vi "Load Table.vi"(4 "XY Graph2":refnum<vi>, 5 "XY Graph1":refnum<vi>, 6 "2 Mics? (F)":bool, 7 "Table Ref":refnum<vi>, 8 "error in (no error)":errorcluster, 9 "Result Cluster":T1, 10 "Config Type":T2={"PSU"={"Current Lower (mA)"=0.0, "Current Upper (mA)"=0.0, "Voltage Lower (V)"=0.0, "Voltage Upper (V)"=0.0}, "Mic"={"Sensitivity (mV/Pa)"={"Lower"=0.0, "Upper"=0.0}, "THD (%)"={"Lower"=0.0, "Upper"=0.0}, "Freq Response"=[]}, "Power Supply"={"Channel Name"="1", "Source Delay (Sec)"=0.5, "Measurement:Sense"=1008, "voltage level"=0.0, "voltage level range"=20.0, "current limit"=0.02, "current limit range"=0.02, "resource name"="PSU"}, "Test Sweep"={"Input Settings"={"IEPE min time to settle [s]"=0.0, "Responce Channel Settings"={"DSA response channel settings"={"coupling"=10045, "enable IEPE excitation"=FALSE, "IEPE current [mA]"=4.0}, "response channel info"={"sensor sensitivity"=1000.0, "engineering units"=1, "dB reference"=1.0, "custom label"="EU", "weighting filter"=0, "pregain"=0.0}, "AI response settings"={"response channel"="SOUNDACQ/ai1", "max value [V]"=10.0, "min value [V]"=-10.0, "terminal configuration"=-1}}, "Stimulus Channel Settings"={"AI stimulus settings"={"stimulus channel"="SOUNDACQ/ai0", "max value [V]"=2.0, "min value [V]"=-2.0, "terminal configuration"=-1}, "DSA stimulus channel settings"={"coupling"=10045, "enable IEPE excitation"=TRUE, "IEPE current [mA]"=4.0}, "stimulus channel info"={"sensor sensitivity"=11.4, "engineering units"=2, "dB reference"=2e-05, "custom label"="EU", "weighting filter"=0, "pregain"=0.0}}}, "Output Settings"={"AO source settings"={"excitation channel"="SOUNDACQ/ao0", "max value [V]"=10.0, "min value [V]"=-10.0, "terminal configuration"=-1}}}} {"Test Sweep"."Output Settings"."AO source settings"."terminal configuration" items=["Default"=-1, "RSE"=10083, "Differential"=10106, "Pseudodifferential"=12529]; "Test Sweep"."Output Settings"."AO source settings"."min value [V]" format="%0.2f"; "Test Sweep"."Output Settings"."AO source settings"."max value [V]" format="%0.2f"; "Test Sweep"."Input Settings"."Stimulus Channel Settings"."stimulus channel info"."pregain" format="%.2f"; "Test Sweep"."Input Settings"."Stimulus Channel Settings"."stimulus channel info"."weighting filter" items=["Linear", "A-weighting", "B-weighting", "C-weighting", "ITU-R 468-4", "Dolby", "CCITT", "C-message", "Wb", "Wc", "Wd", "We", "Wf", "Wh", "Wj", "Wk", "Wm", "AES17 20 kHz lowpass", "AES17 40 kHz lowpass", "AES17 20 kHz highpass", "AES17 40 kHz highpass"]; "Test Sweep"."Input Settings"."Stimulus Channel Settings"."stimulus channel info"."dB reference" format="%^.1e"; "Test Sweep"."Input Settings"."Stimulus Channel Settings"."stimulus channel info"."engineering units" items=["custom..."=0, "V"=1, "A"=21, "C"=30, "pC"=31, "s"=32, "-"=29, "Pa"=2, "N"=20, "g"=3, "m/s^2"=4, "m/s"=5, "m"=6, "mm/s"=12, "mm"=13, "micron/s"=14, "micron"=15, "in/s^2"=7, "in/s"=8, "in"=9, "mil/s"=10, "mil"=11, "rad/s^2"=16, "rad/s"=17, "rad"=18, "deg/s^2"=26, "deg/s"=27, "deg"=28, "RPM"=22, "cycle/s^2"=23, "Hz"=24, "cycle"=25, "strain"=19]; "Test Sweep"."Input Settings"."Stimulus Channel Settings"."stimulus channel info"."sensor sensitivity" format="%#_5f"; "Test Sweep"."Input Settings"."Stimulus Channel Settings"."DSA stimulus channel settings"."IEPE current [mA]" format="%.1f"; "Test Sweep"."Input Settings"."Stimulus Channel Settings"."DSA stimulus channel settings"."coupling" items=["AC"=10045, "DC"=10050, "GND"=10066]; "Test Sweep"."Input Settings"."Stimulus Channel Settings"."AI stimulus settings"."terminal configuration" items=["Default"=-1, "RSE"=10083, "NRSE"=10078, "Differential"=10106, "Pseudodifferential"=12529]; "Test Sweep"."Input Settings"."Stimulus Channel Settings"."AI stimulus settings"."min value [V]" format="%.2f"; "Test Sweep"."Input Settings"."Stimulus Channel Settings"."AI stimulus settings"."max value [V]" format="%.2f"; "Test Sweep"."Input Settings"."Responce Channel Settings"."AI response settings"."terminal configuration" items=["Default"=-1, "RSE"=10083, "NRSE"=10078, "Differential"=10106, "Pseudodifferential"=12529]; "Test Sweep"."Input Settings"."Responce Channel Settings"."AI response settings"."min value [V]" format="%.2f"; "Test Sweep"."Input Settings"."Responce Channel Settings"."AI response settings"."max value [V]" format="%.2f"; "Test Sweep"."Input Settings"."Responce Channel Settings"."response channel info"."pregain" format="%.2f"; "Test Sweep"."Input Settings"."Responce Channel Settings"."response channel info"."weighting filter" items=["Linear", "A-weighting", "B-weighting", "C-weighting", "ITU-R 468-4", "Dolby", "CCITT", "C-message", "Wb", "Wc", "Wd", "We", "Wf", "Wh", "Wj", "Wk", "Wm", "AES17 20 kHz lowpass", "AES17 40 kHz lowpass", "AES17 20 kHz highpass", "AES17 40 kHz highpass"]; "Test Sweep"."Input Settings"."Responce Channel Settings"."response channel info"."dB reference" format="%^.1e"; "Test Sweep"."Input Settings"."Responce Channel Settings"."response channel info"."engineering units" items=["custom..."=0, "V"=1, "A"=21, "C"=30, "pC"=31, "s"=32, "-"=29, "Pa"=2, "N"=20, "g"=3, "m/s^2"=4, "m/s"=5, "m"=6, "mm/s"=12, "mm"=13, "micron/s"=14, "micron"=15, "in/s^2"=7, "in/s"=8, "in"=9, "mil/s"=10, "mil"=11, "rad/s^2"=16, "rad/s"=17, "rad"=18, "deg/s^2"=26, "deg/s"=27, "deg"=28, "RPM"=22, "cycle/s^2"=23, "Hz"=24, "cycle"=25, "strain"=19]; "Test Sweep"."Input Settings"."Responce Channel Settings"."response channel info"."sensor sensitivity" format="%#_5f"; "Test Sweep"."Input Settings"."Responce Channel Settings"."DSA response channel settings"."IEPE current [mA]" format="%.1f"; "Test Sweep"."Input Settings"."Responce Channel Settings"."DSA response channel settings"."coupling" items=["AC"=10045, "DC"=10050, "GND"=10066]; "Test Sweep"."Input Settings"."IEPE min time to settle [s]" format="%.1f"; "Power Supply"."current limit range" format="%_6p"; "Power Supply"."current limit" format="%_6p"; "Power Supply"."voltage level range" format="%_6p"; "Power Supply"."voltage level" format="%_6p"; "Power Supply"."Measurement:Sense" items=["Local"=1008, "Remote"=1009]; "Power Supply"."Source Delay (Sec)" format="%_6p"}, 11 "Freq List In":cluster{"Freq":dbl, "Amp":dbl}[](array[cluster])) -> (0 "error out":errorcluster, 1 "Result Cluster Out":T1, 2 "Table":string[][](table), 3 "Config Type Out":T2={"PSU"={"Current Lower (mA)"=0.0, "Current Upper (mA)"=0.0, "Voltage Lower (V)"=0.0, "Voltage Upper (V)"=0.0}, "Mic"={"Sensitivity (mV/Pa)"={"Lower"=0.0, "Upper"=0.0}, "THD (%)"={"Lower"=0.0, "Upper"=0.0}, "Freq Response"=[]}, "Power Supply"={"Channel Name"="1", "Source Delay (Sec)"=0.5, "Measurement:Sense"=1008, "voltage level"=0.0, "voltage level range"=20.0, "current limit"=0.02, "current limit range"=0.02, "resource name"="PSU"}, "Test Sweep"={"Input Settings"={"IEPE min time to settle [s]"=0.0, "Responce Channel Settings"={"DSA response channel settings"={"coupling"=10045, "enable IEPE excitation"=FALSE, "IEPE current [mA]"=4.0}, "response channel info"={"sensor sensitivity"=1000.0, "engineering units"=1, "dB reference"=1.0, "custom label"="EU", "weighting filter"=0, "pregain"=0.0}, "AI response settings"={"response channel"="SOUNDACQ/ai1", "max value [V]"=10.0, "min value [V]"=-10.0, "terminal configuration"=-1}}, "Stimulus Channel Settings"={"AI stimulus settings"={"stimulus channel"="SOUNDACQ/ai0", "max value [V]"=2.0, "min value [V]"=-2.0, "terminal configuration"=-1}, "DSA stimulus channel settings"={"coupling"=10045, "enable IEPE excitation"=TRUE, "IEPE current [mA]"=4.0}, "stimulus channel info"={"sensor sensitivity"=11.4, "engineering units"=2, "dB reference"=2e-05, "custom label"="EU", "weighting filter"=0, "pregain"=0.0}}}, "Output Settings"={"AO source settings"={"excitation channel"="SOUNDACQ/ao0", "max value [V]"=10.0, "min value [V]"=-10.0, "terminal configuration"=-1}}}} {"Test Sweep"."Output Settings"."AO source settings"."terminal configuration" items=["Default"=-1, "RSE"=10083, "Differential"=10106, "Pseudodifferential"=12529]; "Test Sweep"."Output Settings"."AO source settings"."min value [V]" format="%0.2f"; "Test Sweep"."Output Settings"."AO source settings"."max value [V]" format="%0.2f"; "Test Sweep"."Input Settings"."Stimulus Channel Settings"."stimulus channel info"."pregain" format="%.2f"; "Test Sweep"."Input Settings"."Stimulus Channel Settings"."stimulus channel info"."weighting filter" items=["Linear", "A-weighting", "B-weighting", "C-weighting", "ITU-R 468-4", "Dolby", "CCITT", "C-message", "Wb", "Wc", "Wd", "We", "Wf", "Wh", "Wj", "Wk", "Wm", "AES17 20 kHz lowpass", "AES17 40 kHz lowpass", "AES17 20 kHz highpass", "AES17 40 kHz highpass"]; "Test Sweep"."Input Settings"."Stimulus Channel Settings"."stimulus channel info"."dB reference" format="%^.1e"; "Test Sweep"."Input Settings"."Stimulus Channel Settings"."stimulus channel info"."engineering units" items=["custom..."=0, "V"=1, "A"=21, "C"=30, "pC"=31, "s"=32, "-"=29, "Pa"=2, "N"=20, "g"=3, "m/s^2"=4, "m/s"=5, "m"=6, "mm/s"=12, "mm"=13, "micron/s"=14, "micron"=15, "in/s^2"=7, "in/s"=8, "in"=9, "mil/s"=10, "mil"=11, "rad/s^2"=16, "rad/s"=17, "rad"=18, "deg/s^2"=26, "deg/s"=27, "deg"=28, "RPM"=22, "cycle/s^2"=23, "Hz"=24, "cycle"=25, "strain"=19]; "Test Sweep"."Input Settings"."Stimulus Channel Settings"."stimulus channel info"."sensor sensitivity" format="%#_5f"; "Test Sweep"."Input Settings"."Stimulus Channel Settings"."DSA stimulus channel settings"."IEPE current [mA]" format="%.1f"; "Test Sweep"."Input Settings"."Stimulus Channel Settings"."DSA stimulus channel settings"."coupling" items=["AC"=10045, "DC"=10050, "GND"=10066]; "Test Sweep"."Input Settings"."Stimulus Channel Settings"."AI stimulus settings"."terminal configuration" items=["Default"=-1, "RSE"=10083, "NRSE"=10078, "Differential"=10106, "Pseudodifferential"=12529]; "Test Sweep"."Input Settings"."Stimulus Channel Settings"."AI stimulus settings"."min value [V]" format="%.2f"; "Test Sweep"."Input Settings"."Stimulus Channel Settings"."AI stimulus settings"."max value [V]" format="%.2f"; "Test Sweep"."Input Settings"."Responce Channel Settings"."AI response settings"."terminal configuration" items=["Default"=-1, "RSE"=10083, "NRSE"=10078, "Differential"=10106, "Pseudodifferential"=12529]; "Test Sweep"."Input Settings"."Responce Channel Settings"."AI response settings"."min value [V]" format="%.2f"; "Test Sweep"."Input Settings"."Responce Channel Settings"."AI response settings"."max value [V]" format="%.2f"; "Test Sweep"."Input Settings"."Responce Channel Settings"."response channel info"."pregain" format="%.2f"; "Test Sweep"."Input Settings"."Responce Channel Settings"."response channel info"."weighting filter" items=["Linear", "A-weighting", "B-weighting", "C-weighting", "ITU-R 468-4", "Dolby", "CCITT", "C-message", "Wb", "Wc", "Wd", "We", "Wf", "Wh", "Wj", "Wk", "Wm", "AES17 20 kHz lowpass", "AES17 40 kHz lowpass", "AES17 20 kHz highpass", "AES17 40 kHz highpass"]; "Test Sweep"."Input Settings"."Responce Channel Settings"."response channel info"."dB reference" format="%^.1e"; "Test Sweep"."Input Settings"."Responce Channel Settings"."response channel info"."engineering units" items=["custom..."=0, "V"=1, "A"=21, "C"=30, "pC"=31, "s"=32, "-"=29, "Pa"=2, "N"=20, "g"=3, "m/s^2"=4, "m/s"=5, "m"=6, "mm/s"=12, "mm"=13, "micron/s"=14, "micron"=15, "in/s^2"=7, "in/s"=8, "in"=9, "mil/s"=10, "mil"=11, "rad/s^2"=16, "rad/s"=17, "rad"=18, "deg/s^2"=26, "deg/s"=27, "deg"=28, "RPM"=22, "cycle/s^2"=23, "Hz"=24, "cycle"=25, "strain"=19]; "Test Sweep"."Input Settings"."Responce Channel Settings"."response channel info"."sensor sensitivity" format="%#_5f"; "Test Sweep"."Input Settings"."Responce Channel Settings"."DSA response channel settings"."IEPE current [mA]" format="%.1f"; "Test Sweep"."Input Settings"."Responce Channel Settings"."DSA response channel settings"."coupling" items=["AC"=10045, "DC"=10050, "GND"=10066]; "Test Sweep"."Input Settings"."IEPE min time to settle [s]" format="%.1f"; "Power Supply"."current limit range" format="%_6p"; "Power Supply"."current limit" format="%_6p"; "Power Supply"."voltage level range" format="%_6p"; "Power Supply"."voltage level" format="%_6p"; "Power Supply"."Measurement:Sense" items=["Local"=1008, "Remote"=1009]; "Power Supply"."Source Delay (Sec)" format="%_6p"})   [LabVIEW 2018]
uses:
  Types/ME79 Specs.ctl
  <vilib>/addons/_NISVFA/_Shared subVIs/Controls/svc_DSA Channel Settings.ctl
  <vilib>/addons/_NISVFA/_Shared subVIs/Controls/svc_Channel Info.ctl
  <vilib>/addons/_NISVFA/_Shared subVIs/Controls/svc_Engineering Units Text Ring.ctl
  <vilib>/addons/_NISVFA/_Shared subVIs/Controls/svc_Weighting Filter Text Ring.ctl
  Types/Test Data Type.ctl
panel:
  # "Power Supply"
  # "Power Supply"
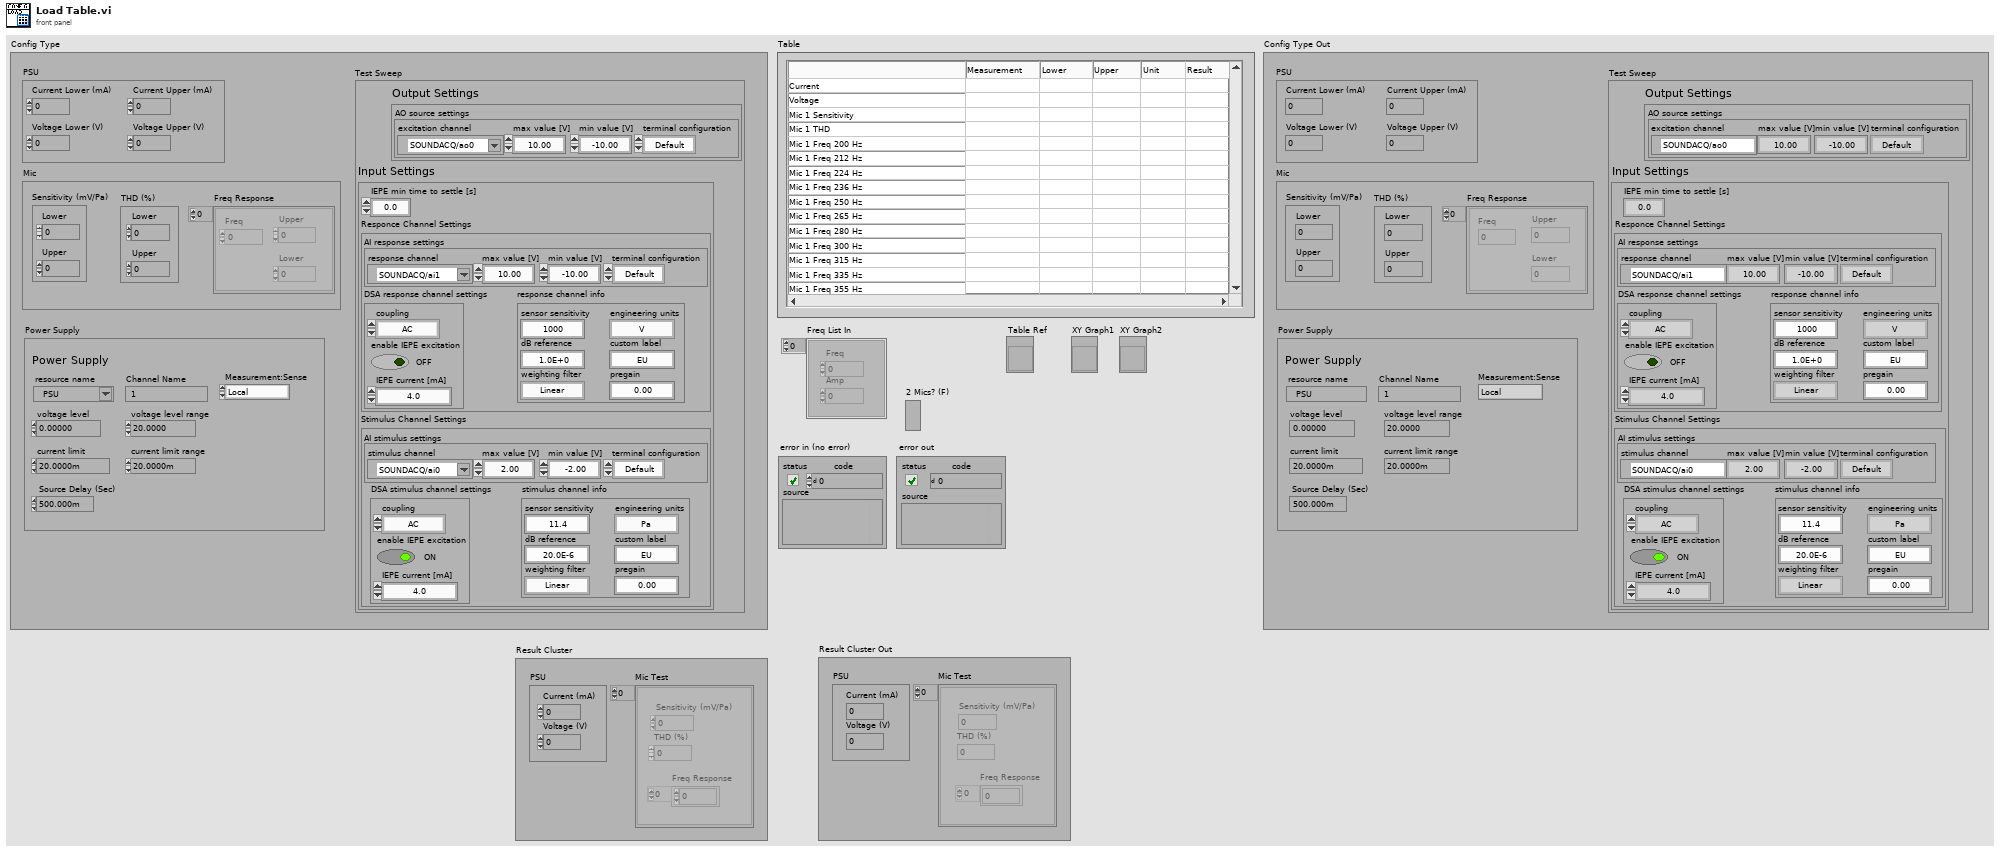
[diagram p1: front panel]
types:
  T1 = typedef "Test Data Type.ctl" = cluster{"PSU":cluster{"Current (mA)":dbl, "Voltage (V)":dbl}, "Mic Test":cluster{"Sensitivity (mV/Pa)":dbl, "THD (%)":dbl, "Freq Response":dbl[]}[]}
  T2 = typedef "ME79 Specs.ctl" = cluster{"PSU":cluster{"Current Lower (mA)":dbl, "Current Upper (mA)":dbl, "Voltage Lower (V)":dbl, "Voltage Upper (V)":dbl}, "Mic":cluster{"Sensitivity (mV/Pa)":cluster{"Lower":dbl, "Upper":dbl}, "THD (%)":cluster{"Lower":dbl, "Upper":dbl}, "Freq Response":cluster{"Freq":dbl, "Upper":dbl, "Lower":dbl}[]}, "Power Supply":cluster{"Channel Name":string, "Source Delay (Sec)":dbl, "Measurement:Sense":i32, "voltage level":dbl, "voltage level range":dbl, "current limit":dbl, "current limit range":dbl, "resource name":refnum<k15>}, "Test Sweep":cluster{"Input Settings":cluster{"IEPE min time to settle [s]":dbl, "Responce Channel Settings":cluster{"DSA response channel settings":T3, "response channel info":T4, "AI response settings":cluster{"response channel":tag, "max value [V]":dbl, "min value [V]":dbl, "terminal configuration":i32}}, "Stimulus Channel Settings":cluster{"AI stimulus settings":cluster{"stimulus channel":tag, "max value [V]":dbl, "min value [V]":dbl, "terminal configuration":i32}, "DSA stimulus channel settings":T3, "stimulus channel info":T4}}, "Output Settings":cluster{"AO source settings":cluster{"excitation channel":tag, "max value [V]":dbl, "min value [V]":dbl, "terminal configuration":i32}}}}
  T3 = typedef "svc_DSA Channel Settings.ctl" = cluster{"coupling":i32, "enable IEPE excitation":bool, "IEPE current [mA]":dbl}
  T4 = typedef "svc_Channel Info.ctl" = cluster{"sensor sensitivity":dbl, "engineering units":T5, "dB reference":dbl, "custom label":string, "weighting filter":T6, "pregain":dbl}
  T5 = typedef "svc_Engineering Units Text Ring.ctl" = u16
  T6 = typedef "svc_Weighting Filter Text Ring.ctl" = u16
  T7 = cluster{"Sensitivity (mV/Pa)":dbl, "THD (%)":dbl, "Freq Response":dbl[]}[]
  T8 = cluster{"Sensitivity (mV/Pa)":dbl, "THD (%)":dbl, "Freq Response":dbl[]}
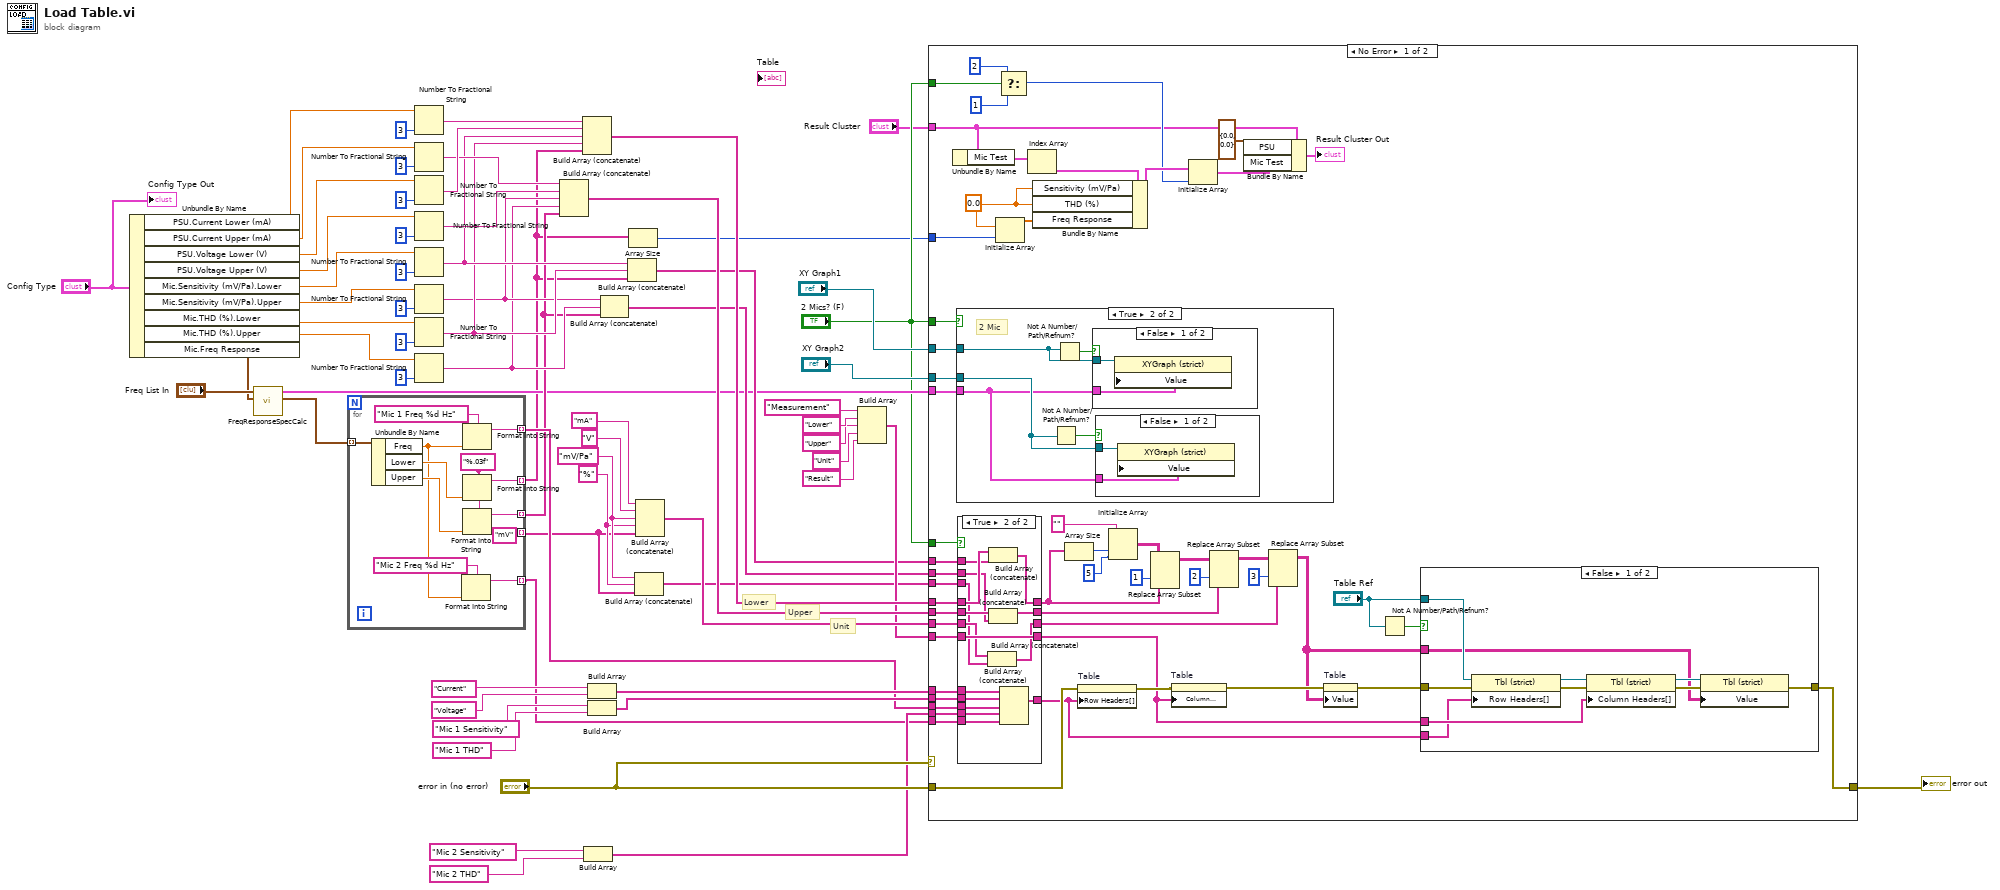
[diagram p0: block diagram]
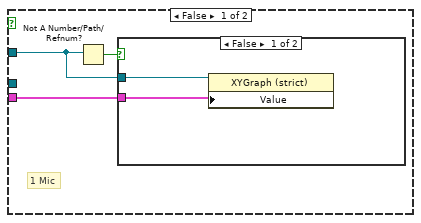
[diagram p2: hidden frame]
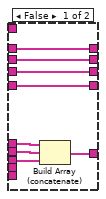
[diagram p7: hidden frame]
diagram:
  w19 = "%"
  w20 = "mV/Pa"
  # "Unit"
  # "Upper"
  # "Lower"
  n1 = Unbundle By Name("Config Type") -> ("PSU.Current Lower (mA)"=w60:dbl, "PSU.Current Upper (mA)"=w50:dbl, "PSU.Voltage Lower (V)"=w49:dbl, "PSU.Voltage Upper (V)"=w48:dbl, "Mic.Sensitivity (mV/Pa).Lower"=w47:dbl, "Mic.Sensitivity (mV/Pa).Upper"=w46:dbl, "Mic.THD (%).Lower"=w45:dbl, "Mic.THD (%).Upper"=w44:dbl, "Mic.Freq Response"=w10:cluster{"Freq":dbl, "Upper":dbl, "Lower":dbl}[])
  n2 = call "FreqResponseSpecCalc.vi"("Freq Response"=w10, "Freq List In"="Freq List In") -> ("Freq Response Spec Out"=w9:cluster{"Freq":dbl, "Upper":dbl, "Lower":dbl}[], "XY Graph"=w7:cluster{dbl[], dbl[]}[])  [unwired: 8 in]
  n3 = for {
    tunnel: w9 -> [w78] mode=indexing
    tunnel: [w76] -> w27 mode=indexing
    tunnel: [w72] -> w2 mode=indexing
    tunnel: [w71] -> w17 mode=indexing
    tunnel: ["mV"] -> w18 mode=indexing
    tunnel: [w67] -> w12 mode=indexing
    w75 = "%.03f"
    n4 = Unbundle By Name(w78) -> ("Freq"=w68:dbl, "Lower"=w74:dbl, "Upper"=w73:dbl)
    n5 = Format Into String(format string="Mic 2 Freq %d Hz", w68) -> (resulting string=w67:string)  [unwired: 2 in, 1 out]
    n6 = Format Into String(format string="Mic 1 Freq %d Hz", w68) -> (resulting string=w76:string)  [unwired: 2 in, 1 out]
    n7 = Format Into String(format string=w75, w74) -> (resulting string=w72:string)  [unwired: 2 in, 1 out]
    n8 = Format Into String(format string=w75, w73) -> (resulting string=w71:string)  [unwired: 2 in, 1 out]
  }
  n9 = Number To Fractional String(number=w60, precision (6)=i16 3) -> (F-format string=w58:string)  [unwired: 2 in]
  n10 = Number To Fractional String(number=w50, precision (6)=i16 3) -> (F-format string=w42:string)  [unwired: 2 in]
  n11 = Number To Fractional String(number=w49, precision (6)=i16 3) -> (F-format string=w43:string)  [unwired: 2 in]
  n12 = Number To Fractional String(number=w48, precision (6)=i16 3) -> (F-format string=w41:string)  [unwired: 2 in]
  n13 = Number To Fractional String(number=w47, precision (6)=i16 3) -> (F-format string=w26:string)  [unwired: 2 in]
  n14 = Number To Fractional String(number=w46, precision (6)=i16 3) -> (F-format string=w24:string)  [unwired: 2 in]
  n15 = Number To Fractional String(number=w45, precision (6)=i16 3) -> (F-format string=w25:string)  [unwired: 2 in]
  n16 = Number To Fractional String(number=w44, precision (6)=i16 3) -> (F-format string=w23:string)  [unwired: 2 in]
  n17 = Build Array (concatenate)(w42, w41, w24, w23, w17) -> (w40:string[])
  n18 = Build Array (concatenate)(w58, w43, w26, w25, w2) -> (w39:string[])
  n19 = Build Array("Mic 2 Sensitivity", "Mic 2 THD") -> (w13:string[])
  n20 = Build Array("Current", "Voltage") -> (w29:string[])
  n21 = Build Array("Mic 1 Sensitivity", "Mic 1 THD") -> (w28:string[])
  n22 = Build Array (concatenate)(w24, w23, w17) -> (w21:string[])
  n23 = Build Array (concatenate)(w26, w25, w2) -> (w22:string[])
  n24 = Array Size(array=w2) -> (size(s)=w1:i32)
  n25 = Build Array (concatenate)(w20, w19, w18) -> (w16:string[])
  n26 = Build Array (concatenate)("mA", "V", w20, w19, w18) -> (w36:string[])
  n27 = Build Array("Measurement", "Lower", "Upper", "Unit", "Result") -> (w30:string[])
  n28 = case shown="No Error" "error in (no error)" {
    tunnel: "error in (no error)" -> [w131 w181]
    tunnel: [w104 w181] -> w61
    tunnel: w39 -> [w119 _]
    tunnel: w40 -> [w118 _]
    tunnel: w36 -> [w117 _]
    tunnel: w30 -> [w116 _]
    tunnel: w29 -> [w123 _]
    tunnel: "2 Mics? (F)" -> [w122 _]
    tunnel: w28 -> [w121 _]
    tunnel: w27 -> [w120 _]
    tunnel: w22 -> [w113 _]
    tunnel: w21 -> [w112 _]
    tunnel: w16 -> [w111 _]
    tunnel: w13 -> [w98 _]
    tunnel: w12 -> [w97 _]
    tunnel: w7 -> [w94 _]
    tunnel: "2 Mics? (F)" -> [w96 _]
    tunnel: "XY Graph1" -> [w95 _]
    tunnel: "XY Graph2" -> [w93 _]
    tunnel: "2 Mics? (F)" -> [w92 _]
    tunnel: "Result Cluster" -> [w82 _]
    tunnel: w1 -> [w88 _]
    frame No Error {
      w85 = 0.0
      n29 = Unbundle By Name(w82) -> ("Mic Test"=w89:T7)
      n30 = case shown="True" w96 {
        tunnel: w95 -> [w132 w140]
        tunnel: w94 -> [w133 w137]
        tunnel: w93 -> [_ w138]
        frame False {
          # "1 Mic"
          n31 = Not A Number/Path/Refnum?(number/path/refnum=w132) -> (NaN/Path/Refnum?=w134:bool)
          n32 = case shown="False" w134 {
            tunnel: w132 -> [w136 _]
            tunnel: w133 -> [w135 _]
            frame False {
              n33 = property class="XYGraph (strict)"(reference=w136, "Value"=w135) -> ()  [unwired: 1 in, 2 out]
            }
            frame True {
            }
          }
        }
        frame True {
          # "2 Mic"
          n34 = Not A Number/Path/Refnum?(number/path/refnum=w138) -> (NaN/Path/Refnum?=w139:bool)
          n35 = Not A Number/Path/Refnum?(number/path/refnum=w140) -> (NaN/Path/Refnum?=w141:bool)
          n36 = case shown="False" w141 {
            tunnel: w140 -> [w145 _]
            tunnel: w137 -> [w144 _]
            frame False {
              n37 = property class="XYGraph (strict)"(reference=w145, "Value"=w144) -> ()  [unwired: 1 in, 2 out]
            }
            frame True {
            }
          }
          n38 = case shown="False" w139 {
            tunnel: w138 -> [w143 _]
            tunnel: w137 -> [w142 _]
            frame False {
              n39 = property class="XYGraph (strict)"(reference=w143, "Value"=w142) -> ()  [unwired: 1 in, 2 out]
            }
            frame True {
            }
          }
        }
      }
      n40 = case shown="True" w122 {
        tunnel: w123 -> [w164 w180]
        tunnel: w121 -> [w163 w179]
        tunnel: w120 -> [w162 w166]
        tunnel: [w161 w178] -> w107
        tunnel: w119 -> [w160 w177]
        tunnel: w118 -> [w159 w173]
        tunnel: w117 -> [w158 w170]
        tunnel: w116 -> [w157 w174]
        tunnel: [w160 w175] -> w102
        tunnel: [w159 w171] -> w115
        tunnel: [w158 w168] -> w114
        tunnel: [w157 w174] -> w106
        tunnel: w113 -> [_ w176]
        tunnel: w112 -> [_ w172]
        tunnel: w111 -> [_ w169]
        tunnel: w98 -> [_ w167]
        tunnel: w97 -> [_ w165]
        frame False {
          n41 = Build Array (concatenate)(w164, w163, w162) -> (w161:string[])
        }
        frame True {
          n42 = Build Array (concatenate)(w170, w169) -> (w168:string[])
          n43 = Build Array (concatenate)(w177, w176) -> (w175:string[])
          n44 = Build Array (concatenate)(w173, w172) -> (w171:string[])
          n45 = Build Array (concatenate)(w180, w179, w166, w167, w165) -> (w178:string[])
        }
      }
      n46 = Initialize Array(w85, w88) -> (w86:dbl[])
      n47 = Select(t=2, s=w92, f=1) -> (s? t:f=w83:i32)
      n48 = Index Array(array=w89) -> (element=w87:T8)  [unwired: 1 in]
      n49 = Bundle By Name(cluster=w87, "Sensitivity (mV/Pa)"=w85, "THD (%)"=w85, "Freq Response"=w86) -> (w84:T8)
      n50 = Array Size(array=w102) -> (size(s)=w100:i32)
      n51 = property on="Table" class="Tbl (strict)"(error in=w131, "Row Headers[]"=w107) -> (error out=w125:errorcluster)  [unwired: 1 in, 1 out]
      n52 = Initialize Array("", w100, 5 ("dimension size")) -> (w101:string[][])
      n53 = Replace Array Subset(array=w101, new element=w102, index (col)=1 ("disabled index (col)")) -> (w129:string[][])  [unwired: 1 in]
      n54 = property on="Table" class="Tbl (strict)"(error in=w125, "Column Headers[]"=w106) -> (error out=w124:errorcluster)  [unwired: 1 in, 1 out]
      n55 = Initialize Array(w84, w83) -> (w81:T7)
      n56 = Replace Array Subset(array=w129, new element=w115, index (col)=2 ("disabled index (col)")) -> (w126:string[][])  [unwired: 1 in]
      n57 = Bundle By Name(cluster=w82, "PSU"=cluster{"Current (mA)":dbl, "Voltage (V)":dbl} {"Current (mA)"=0.0, "Voltage (V)"=0.0}, "Mic Test"=w81) -> (→"Result Cluster Out":T1)
      n58 = Replace Array Subset(array=w126, new element=w114, index (col)=3 ("disabled index (col)")) -> (w105:string[][])  [unwired: 1 in]
      n59 = property on="Table" class="Tbl (strict)"(error in=w124, "Value"=w105) -> (error out=w108:errorcluster)  [unwired: 1 in, 1 out]
      n60 = Not A Number/Path/Refnum?(number/path/refnum="Table Ref") -> (NaN/Path/Refnum?=w110:bool)
      n61 = case shown="False" w110 {
        tunnel: "Table Ref" -> [w155 _]
        tunnel: w108 -> [w154 w156]
        tunnel: w107 -> [w147 _]
        tunnel: w106 -> [w148 _]
        tunnel: w105 -> [w149 _]
        tunnel: [w146 w156] -> w104
        frame False {
          n62 = property class="Tbl (strict)"(reference=w155, error in=w154, "Row Headers[]"=w147) -> (reference out=w153:refnum<vi>, error out=w152:errorcluster)
          n63 = property class="Tbl (strict)"(reference=w153, error in=w152, "Column Headers[]"=w148) -> (reference out=w151:refnum<vi>, error out=w150:errorcluster)
          n64 = property class="Tbl (strict)"(reference=w151, error in=w150, "Value"=w149) -> (error out=w146:errorcluster)  [unwired: 1 out]
        }
        frame True {
        }
      }
    }
    frame Error {
    }
  }
  "error out" <- w61
  "Config Type Out" <- "Config Type"
